vi "makePathLocal.vi"(10 "storedPath":path) -> (2 "loadPath":path)   [LabVIEW 2022 SP3]
uses:
  Anemometry Sub Vis/Globals/Constants_global.vi
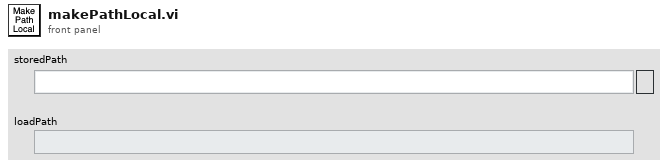
[diagram p1: front panel]
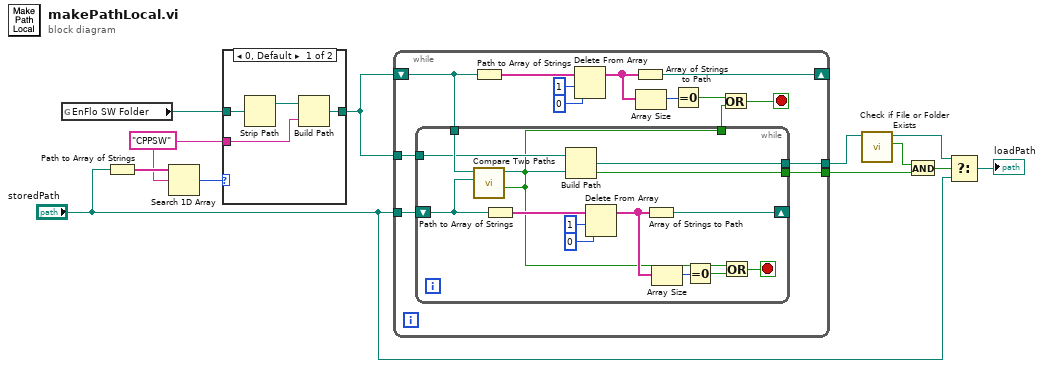
[diagram p0: block diagram]
diagram:
  w1 = "CPPSW" ("element")
  n1 = global read "Constants_global.vi" "EnFlo SW Folder"() -> (w2:path)
  n2 = Path to Array of Strings(0:"storedPath") -> (2:w5:string[])  [unwired: 1 out]
  n3 = Search 1D Array(1D array=w5, element=w1) -> (index of element=w4:i32)  [unwired: 1 in]
  n4 = case shown="0, Default" w4 {
    tunnel: [w15 w17] -> w3
    tunnel: w2 -> [w16 w17]
    tunnel: w1 -> [w13 _]
    frame 0, Default {
      n5 = Strip Path(path=w16) -> (stripped path=w14:path)  [unwired: 1 out]
      n6 = Build Path(base path=w14, name or relative path=w13) -> (appended path=w15:path)
    }
    frame -1 {
    }
  }
  n7 = while {
    tunnel: "storedPath" -> [w31]
    tunnel: [w30] -> w10
    shift-right: [w26] -> _
    shift-left: w3 -> [w25]
    tunnel: w3 -> [w19]
    tunnel: [w18] -> w12
    stop <- w21 stop-if-true
    n8 = while {
      tunnel: w25 -> [w34]
      shift-right: [w40] -> _
      shift-left: w31 -> [w43]
      tunnel: [w35] -> w30 if=w32
      tunnel: [w32] -> w20
      tunnel: w19 -> [w33]
      tunnel: [w32] -> w18
      stop <- w37 stop-if-true
      n9 = call <vilib>:"Compare Two Paths.vi"("Path 2"=w43, "Path 1"=w34) -> ("Path 2 Relative to Path 1?"=w32:bool, "Relative Path from 1 to 2"=w36:path)  [unwired: 6 in, 2 out]
      n10 = Path to Array of Strings(0:w43) -> (2:w39:string[])  [unwired: 1 out]
      n11 = Build Path(base path=w33, name or relative path=w36) -> (appended path=w35:path)
      n12 = Delete From Array(array=w39, length=1, index=0) -> (array with subset deleted=w38:string[])  [unwired: 1 out]
      n13 = Array of Strings to Path(0:w38) -> (2:w40:path)  [unwired: 1 in]
      n14 = Array Size(array=w38) -> (size(s)=w45:i32)
      n15 = Equal To 0?(x=w45) -> (x = 0?=w44:bool)
      n16 = Or(x=w32, y=w44) -> (x .or. y?=w37:bool)
    }
    n17 = Path to Array of Strings(0:w25) -> (2:w27:string[])  [unwired: 1 out]
    n18 = Delete From Array(array=w27, length=1, index=0) -> (array with subset deleted=w23:string[])  [unwired: 1 out]
    n19 = Array of Strings to Path(0:w23) -> (2:w26:path)  [unwired: 1 in]
    n20 = Array Size(array=w23) -> (size(s)=w24:i32)
    n21 = Equal To 0?(x=w24) -> (x = 0?=w22:bool)
    n22 = Or(x=w22, y=w20) -> (x .or. y?=w21:bool)
  }
  n23 = call <vilib>:"Check if File or Folder Exists.vi"("path"=w10) -> ("file or folder exists?"=w7:bool, "dup path"=w9:path)  [unwired: 8 in, 1 out]
  n24 = And(x=w7, y=w12) -> (x .and. y?=w8:bool)
  n25 = Select(t=w9, s=w8, f="storedPath") -> (s? t:f=→"loadPath":path)
